vi "Read Cluster.vi"(8 "error in (no error)":errorcluster, 11 "CallRequest (JSON) in":refnum<class "CallRequest (JSON).lvclass">) -> (0 "error out":errorcluster, 2 "Cluster":T1, 3 "CallRequest (JSON) out":refnum<class "CallRequest (JSON).lvclass">)   [LabVIEW 2020, in "wamplv.lvlib" / "CallRequest (JSON).lvclass"]
uses:
  CallRequest (JSON).lvclass
  TypeDefs/CALL request (JSON).ctl
  WAMP Client/API/TypeDefs/RESULT payload (JSON).ctl
  WAMP Client/API/TypeDefs/Combined error.ctl
  WAMP Client/API/TypeDefs/WAMP error.ctl
  CallRequest (JSON).lvclass/CallRequest (JSON).ctl
  WAMP Client/WAMP Client.lvclass
  wamplv.lvlib
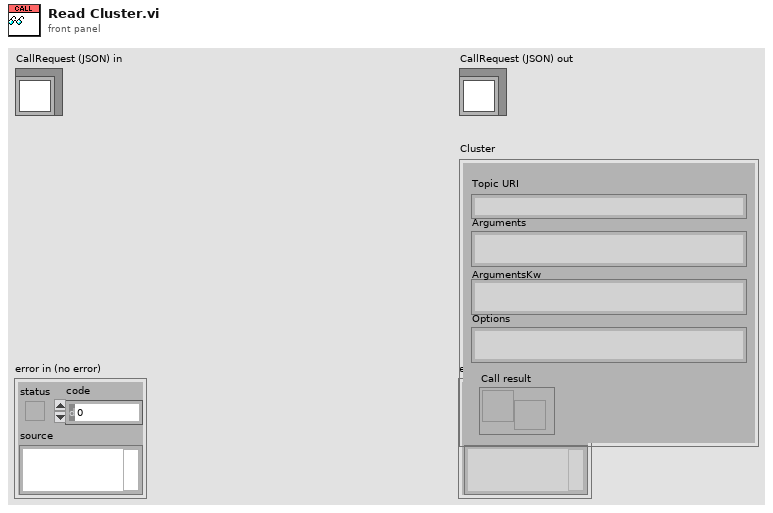
[diagram p1: front panel]
types:
  T1 = typedef "wamplv.lvlib/CALL request (JSON).ctl" = cluster{"Topic URI":string, "Arguments":string, "ArgumentsKw":string, "Options":string, "Call result":refnum<notifier>}
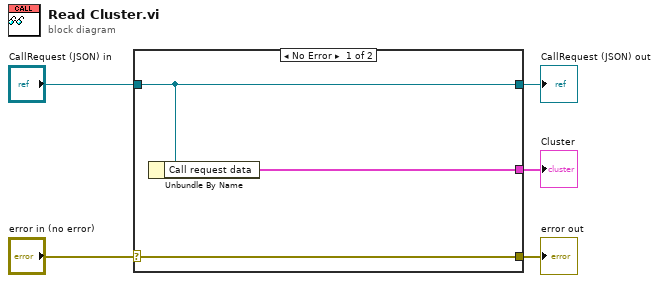
[diagram p0: block diagram]
diagram:
  n1 = case shown="No Error" "error in (no error)" {
    selector: "error in (no error)" -> [w8 w9]
    tunnel: [w8 w9] -> w4
    tunnel: [w7 w10] -> w2
    tunnel: "CallRequest (JSON) in" -> [w7 w10]
    tunnel: [w6 _] -> w1
    frame No Error {
      n2 = Unbundle By Name(w7) -> ("Call request data"=w6:T1)
    }
    frame Error {
    }
  }
  "error out" <- w4
  "CallRequest (JSON) out" <- w2
  "Cluster" <- w1
